vi "Dequeue.vi"(8 "error in (no error)":errorcluster, 11 "PriorityQueue in":refnum<class "PriorityQueue.lvclass">) -> (0 "error out":errorcluster, 1 "Timed Out?":bool, 2 "Element":variant, 3 "PriorityQueue out":refnum<class "PriorityQueue.lvclass">)   [LabVIEW 2019, in "PriorityQueue.lvclass"]
doc: "Dequeues the highest priority element available on the queue. If no elements are available, and empty variant is returned and Timed Out? returns TRUE."
uses:
  PriorityQueue.lvclass
  PriorityQueue.lvclass/PriorityQueue.ctl
panel:
  in  "timeout in ms (-1)":i32
  # "Note: Default implementation does not allow the user to set a timeout value.  Implementing a timeout is shown on the block diagram in the disabled frame."
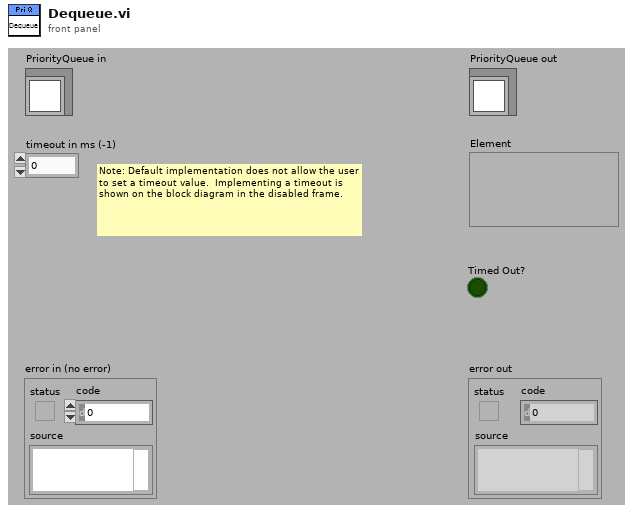
[diagram p1: front panel]
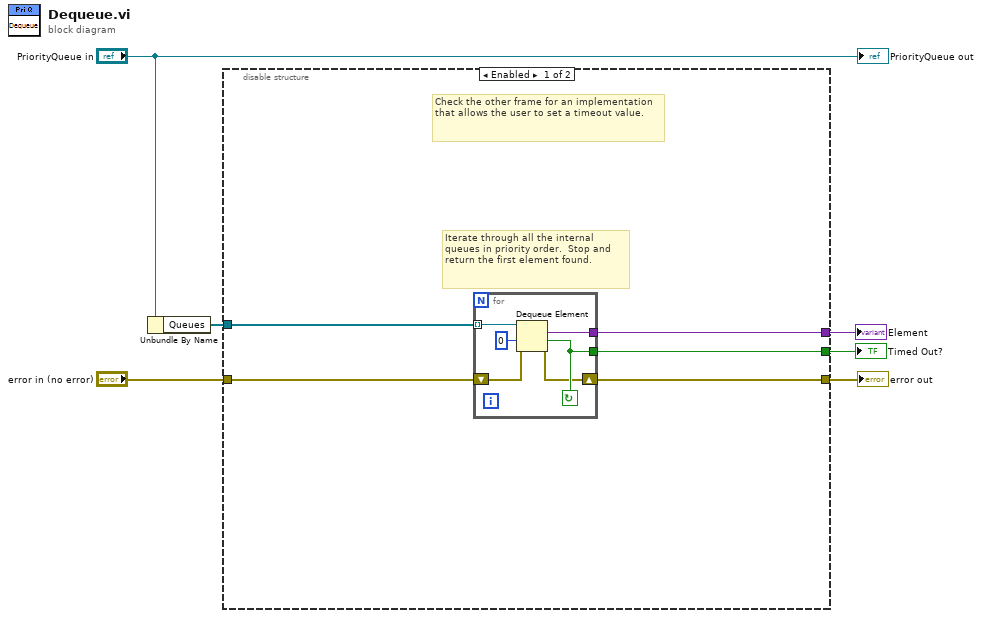
[diagram p0: block diagram]
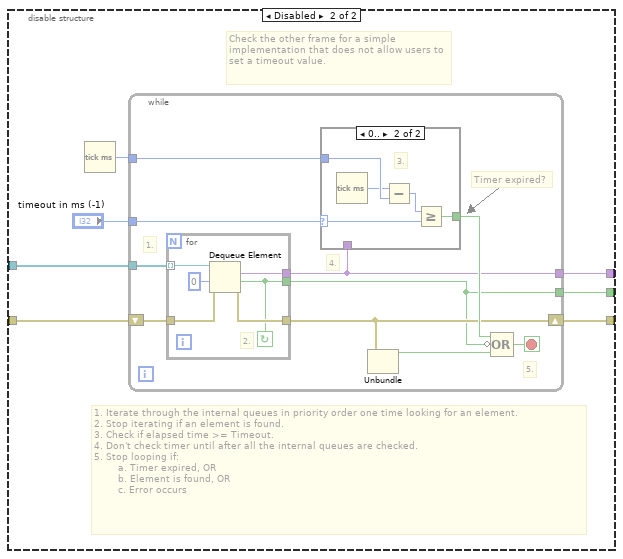
[diagram p2: hidden frame]
diagram:
  n1 = Unbundle By Name("PriorityQueue in") -> ("Queues"=w5:refnum<queue>[])
  n2 = disable-structure shown="Enabled" {
    disable-tunnel: w5 -> [w11 w23]
    disable-tunnel: [w10 w21] -> w4
    disable-tunnel: [w9 w20] -> w3
    disable-tunnel: "error in (no error)" -> [w8 w22]
    disable-tunnel: [w7 w19] -> w1
    frame Enabled {
      # "Check the other frame for an implementation that allows the user to set a timeout value."
      # "Iterate through all the internal queues in priority order.  Stop and return the first element found."
      n3 = for {
        tunnel: w11 -> [w17] mode=indexing
        tunnel: [w16] -> w10
        tunnel: [w15] -> w9
        shift-right: [w13] -> w7
        shift-left: w8 -> [w14]
        stop <- w15 continue-if-true
        n4 = Dequeue Element(queue=w17, timeout in ms (-1)=0, error in (no error)=w14) -> (element=w16:variant, timed out?=w15:bool, error out=w13:errorcluster)  [unwired: 1 out]
      }
    }
    frame Disabled {
      # "1. Iterate through the internal queues in priority order one time looking for an element.\n2. Stop iterating if an element is found.\n3. Check if elapsed time >= Timeout.\n4. Don't check timer until after all the internal queues are checked.\n5. Stop looping if:\n        a. Timer expired, OR\n        b. Element is found, OR\n        c. Error occurs"
      # "Check the other frame for a simple implementation that does not allow users to set a timeout value."
      n5 = Tick Count (ms)() -> (millisecond timer value=w24:u32)
      n6 = while {
        tunnel: w23 -> [w34]
        tunnel: w24 -> [w33]
        tunnel: "timeout in ms (-1)" -> [w32]
        shift-right: [w28] -> w19
        shift-left: w22 -> [w31]
        tunnel: [w25] -> w20
        tunnel: [w27] -> w21
        stop <- w29 stop-if-true
        # "5."
        # "Timer expired?"
        # "4."
        # "1."
        n7 = for {
          tunnel: w34 -> [w45] mode=indexing
          tunnel: [w44] -> w27
          tunnel: [w40] -> w25
          tunnel: w31 -> [w43]
          tunnel: [w42] -> w28
          stop <- w40 continue-if-true
          # "2."
          n8 = Dequeue Element(queue=w45, timeout in ms (-1)=0, error in (no error)=w43) -> (element=w44:variant, timed out?=w40:bool, error out=w42:errorcluster)  [unwired: 1 out]
        }
        n9 = case shown="0.." w32 {
          selector: w32 -> [_ w36]
          tunnel: w33 -> [_ w39]
          tunnel: [_ w35] -> w30
          tunnel: w27 -> [_ _]
          frame ..-1 {
            # "Timer never expires"
          }
          frame 0.. {
            # "3."
            n10 = Tick Count (ms)() -> (millisecond timer value=w38:u32)
            n11 = Subtract(x=w38, y=w39) -> (x-y=w37:u32)
            n12 = Greater Or Equal?(x=w37, y=w36) -> (x >= y?=w35:bool)
          }
        }
        n13 = Unbundle(w28) -> ("status"=w26:bool)  [unwired: 2 out]
        n14 = Compound Arithmetic op=OR(w30, invert w25, w26) -> (w29:bool)
      }
    }
  }
  "error out" <- w1
  "Element" <- w4
  "Timed Out?" <- w3
  "PriorityQueue out" <- "PriorityQueue in"
